vi "Set_Persistent.vi"   [LabVIEW 2019]
uses:
  Instrument_Setup.vi
  Global Variables/Data_Display_global.vi
  Monitors/Utility/Monitor Communication/sub-vis/16T_Open_Queue.vi
  Monitors/Utility/Monitor Communication/sub-vis/16T_Queue_Commands.vi
  Monitors/Utility/Monitor Communication/sub-vis/20T_Open_Queue.vi
  Monitors/Utility/Monitor Communication/sub-vis/20T_Queue_Commands.vi
types:
  T1 = typedef "16T-Cluster.ctl" = cluster{"Clamp":bool, "Switch Heater":bool, "Go to Zero":bool, "Go to set":bool, "Go to Hold":bool, "Clamped":bool, "Quenched":bool, "Rate limit":bool, "Persistent":bool, "Hold":bool, "Set":bool, "Zero":bool, "Magnet (T)":dbl, "Leads (T)":dbl, "Magnet T (K)":dbl, "Switch":bool, "Setpoint (T)":dbl, "Rate (T/min)":dbl, "Select":bool, "Sweeping":bool}
  T2 = typedef "PSIO.ctl" = cluster{"Address":T3, "Version":enum16{"PS", "IPS"}}
  T3 = typedef "OxfordAddress.ctl" = cluster{"Com Port":i32, "ISOBUS Address":i32, "GPIB Address":i16, "Communication":enum16{"RS232", "ISOBUS", "GPIB", "Gateway"}}
  T4 = cluster{"Version\n":string, "Max Sweep(4.2K)":dbl[unit], "Max Sweep(2.2K)":dbl[unit], "Switch htr dly":dbl[unit], "Max Field(4.2K)":dbl[unit], "Max Field(2.2K)":dbl[unit], "Max lead res":dbl[unit], "IO Info":T2}
  T5 = typedef "16T_Control.ctl" = cluster{"Clamp":bool, "Switch Heater":bool, "Go to Zero":bool, "Go to Set":bool, "Go to Hold":bool, "Setpoint (T)":dbl, "Rate (T/min)":dbl, "Set Rate":bool}
  T6 = typedef "15T-Cluster.ctl" = cluster{"Magnet (T)":dbl, "Leads (T)":dbl, "Setpoint (T)":dbl, "Rate (T/min)":dbl, "Set":bool, "Zero":bool, "Hold":bool, "Go to zero":bool, "Go to Hold":bool, "Go to Set":bool, "Clamp":bool, "Switch Heater":bool, "Rate limit":bool, "Switch":bool, "Clamped":bool, "Persistent":bool, "Quenched":bool, "Sweeping":bool, "Select":bool}
  T7 = cluster{"Version\n":string, "Max Sweep":dbl[unit], "Max Field":dbl[unit], "IO Info":T2, "Switch htr dly":dbl[unit]}
  T8 = typedef "15T-Control.ctl" = cluster{"Setpoint (T)":dbl, "Rate (T/min)":dbl, "Go to zero":bool, "Go to Hold":bool, "Go to Set":bool, "Clamp":bool, "Switch Heater":bool}
  T9 = typedef "20T_Cluster.ctl" = cluster{"Clamp":bool, "Switch Heater":bool, "Go to Zero":bool, "Go to set":bool, "Go to Hold":bool, "Clamped":bool, "Hold":bool, "Set":bool, "Zero":bool, "Magnet (T)":dbl, "Leads (T)":dbl, "Magnet T (K)":dbl, "Switch":bool, "Target Field (T)":dbl, "Field Setpoint (T)":dbl, "Rate Setpoint (T/min)":dbl, "Set Rate":bool, "Rate\n(T/min) ":dbl, "lambda NV (%)":dbl, "lambda p (mbar)":dbl, "lambda-Control":bool, "Activate lambda control":bool, "lambda NV  SP":dbl, "Set lambda NV":bool, "PSU Status":string, "PSU\nVoltage":dbl}
  T10 = typedef "20T_Control.ctl" = cluster{"Clamp":bool, "Switch Heater":bool, "Go to Zero":bool, "Go to Set":bool, "Go to Hold":bool, "Field Setpoint (T)":dbl, "Rate Setpoint (T/min)":dbl, "Set Rate":bool, "Activate lambda control":bool, "Set lambda NV":bool, "lambda NV  SP":dbl}
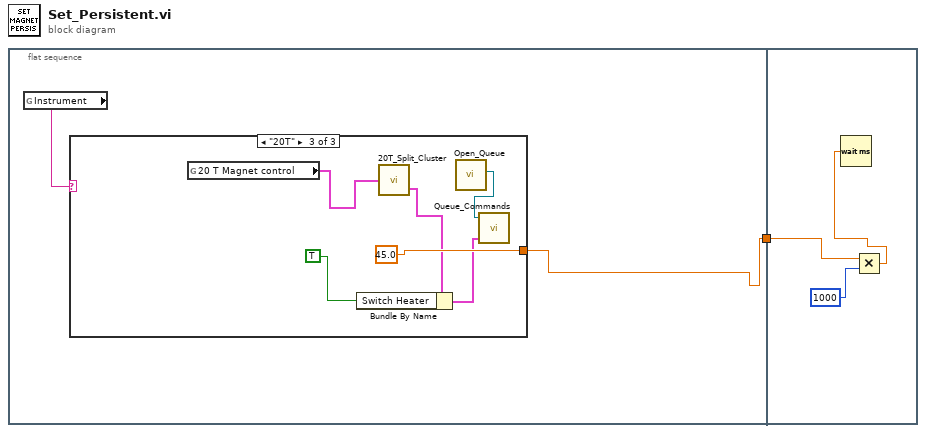
[diagram p0: block diagram]
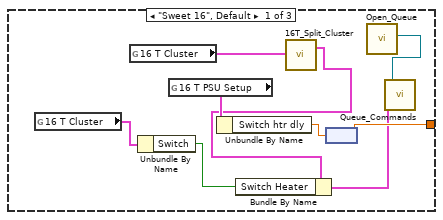
[diagram p2: hidden frame]
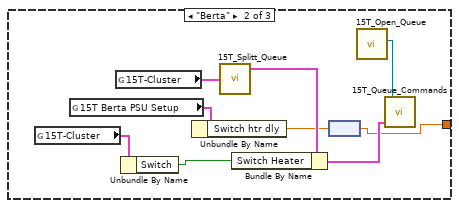
[diagram p3: hidden frame]
diagram:
  n1 = flat-sequence {
    tunnel: [w2] -> w1
    tunnel: w1 -> [w28]
    frame #0 {
      n2 = global read "Instrument_Setup.vi" "Instrument"() -> (w3:string)
      n3 = case shown="\"20T\"" w3 {
        tunnel: [w10 w13 45.0] -> w2
        frame "Sweet 16", Default {
          n4 = global read "Data_Display_global.vi" "16 T Cluster"() -> (w9:T1)
          n5 = global read "Data_Display_global.vi" "16 T Cluster"() -> (w5:T1)
          n6 = Unbundle By Name(w9) -> ("Switch"=w8:bool)
          n7 = global read "Instrument_Setup.vi" "16 T PSU Setup"() -> (w12:T4)
          n8 = Unbundle By Name(w12) -> ("Switch htr dly"=w11:dbl[unit])
          n9 = call "16T_Split_Cluster.vi"("16 T Magnet control"=w5) -> ("16 T Magnet control"=w4:T5)  [unwired: 1 out]
          n10 = Bundle By Name(cluster=w4, "Switch Heater"=w8) -> (w6:T5)
          n11 = node(w11) -> (w10:dbl)
          n12 = call-poly "Open_Queue.vi"() -> ("queue out"=w7:refnum<queue>)  [unwired: 10 in, 1 out]
          n13 = call-poly "Queue_Commands.vi"("16 T Magnet control"=w6, "16T Queue"=w7) -> ()  [unwired: 1 in, 1 out]
        }
        frame "Berta" {
          n14 = global read "Data_Display_global.vi" "15T-Cluster"() -> (w21:T6)
          n15 = global read "Instrument_Setup.vi" "15T Berta PSU Setup"() -> (w15:T7)
          n16 = global read "Data_Display_global.vi" "15T-Cluster"() -> (w20:T6)
          n17 = Unbundle By Name(w21) -> ("Switch"=w18:bool)
          n18 = Unbundle By Name(w15) -> ("Switch htr dly"=w14:dbl[unit])
          n19 = call "15T_Splitt_Queue.vi"("15T-Cluster"=w20) -> ("15T-Control"=w19:T8)  [unwired: 1 in, 1 out]
          n20 = Bundle By Name(cluster=w19, "Switch Heater"=w18) -> (w16:T8)
          n21 = node(w14) -> (w13:dbl)
          n22 = call "15T_Open_Queue.vi"() -> ("queue out"=w17:refnum<queue>)  [unwired: 10 in, 1 out]
          n23 = call "15T_Queue_Commands.vi"("15T-Control"=w16, "15T Queue"=w17) -> ()  [unwired: 1 in, 1 out]
        }
        frame "20T" {
          n24 = global read "Data_Display_global.vi" "20 T Magnet control"() -> (w23:T9)
          n25 = call "20T_Split_Cluster.vi"("20 T Cluster"=w23) -> ("20 T Control"=w22:T10)  [unwired: 1 out]
          n26 = Bundle By Name(cluster=w22, "Switch Heater"=TRUE) -> (w24:T10)
          n27 = call-poly "Open_Queue.vi"() -> ("queue out"=w25:refnum<queue>)  [unwired: 10 in, 1 out]
          n28 = call-poly "Queue_Commands.vi"("20T Control (in)"=w24, "20T Queue"=w25) -> ()  [unwired: 1 in, 1 out]
        }
      }
    }
    frame #1 {
      n29 = Multiply(x=w28, y=1000) -> (x*y=w29:dbl)
      n30 = Wait (ms)(milliseconds to wait=w29) -> ()  [unwired: 1 out]
    }
  }
